vi "Test Initiate.vi"(0 "niDTS BT Rx Test in":refnum<class "niDTS BT Rx Test.lvclass">, 11 "error in (no error)":errorcluster) -> (4 "niDTS BT Rx Test out":refnum<class "niDTS BT Rx Test.lvclass">, 15 "error out":errorcluster)   [LabVIEW 2015, in "niDTS BT.lvlib" / "niDTS BT Rx Test.lvclass"]
uses:
  niDTS BT Rx Test.lvclass
  niDTS BT Rx Test.lvclass/niDTS BT Rx Test.ctl
  Instrument/INSTR RX/niDTS BT INSTR RX.lvclass
  Framework/Dut/Objects/BASE_class/niDTS Dut.lvclass
  Dut/Objects/BASE_class/niDTS BT Dut.lvclass
  niDTS BT.lvlib
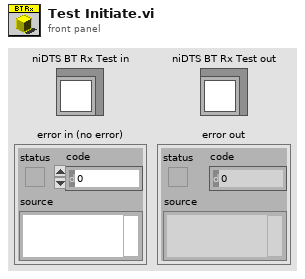
[diagram p1: front panel]
types:
  T1 = typedef "niDTS Framework.lvlib/niDTS Dut INC Handle.ctl" = refnum<data-value>
  T2 = typedef "niDTS BT.lvlib/niDTS BT INC Packet Type.ctl" = enum16{"NULL", "POLL", "FHS", "DM1", "DH1", "HV1", "HV2", "HV3", "EV3", "DV", "AUX1", "DM3", "DH3", "EV4", "EV5", "DM5", "DH5", "LE-TP"}
  T3 = typedef "niDTS BT.lvlib/niDTS BT Dut INC Handle.ctl" = refnum<data-value>
  T4 = typedef "niDTS BT.lvlib/niDTS BT Rx Test INC Results.ctl" = cluster{"Total Packets Received (LE)":i32, "Packets Sent (LE)":dbl, "Good Packets":dbl, "Packet Error Rate (%)":dbl, "Error Bits":u32, "Good Bits":u32, "Total Received Bits":u32, "Bit Error Rate (%)":dbl}
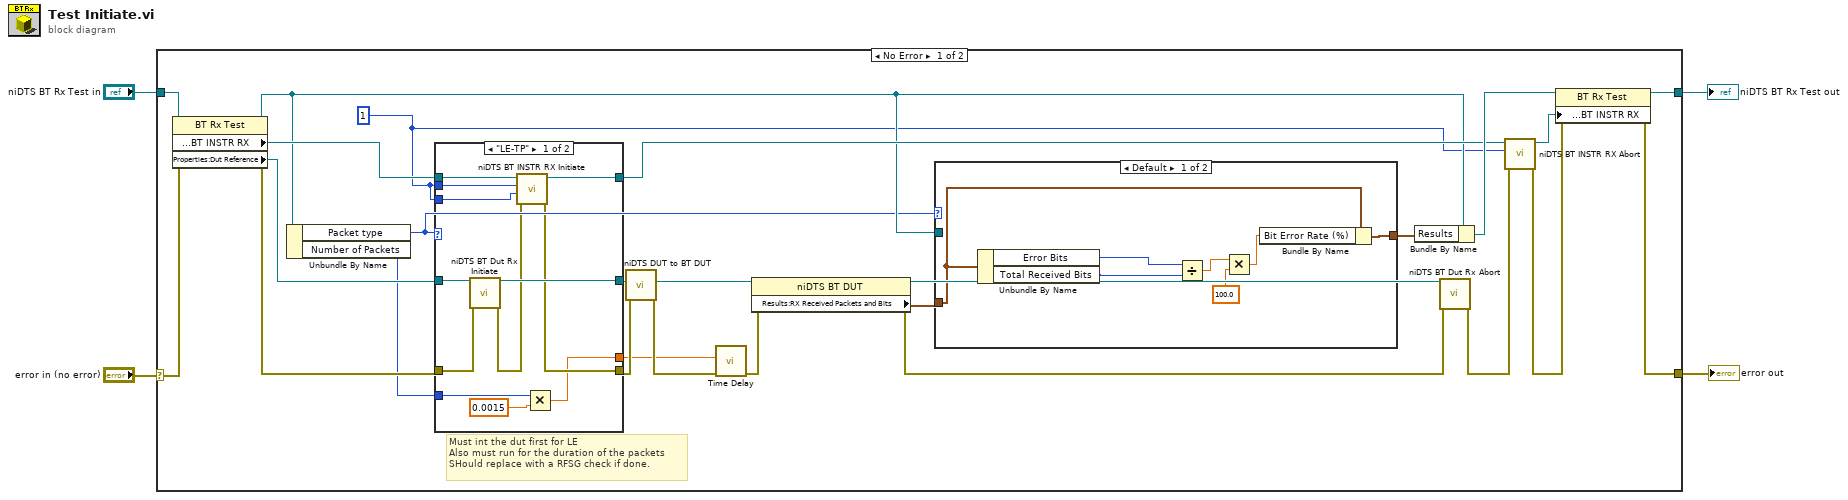
[diagram p0: block diagram]
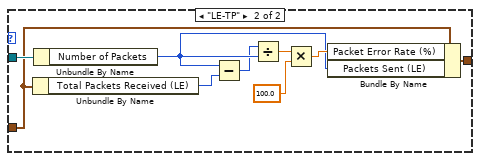
[diagram p2: hidden frame]
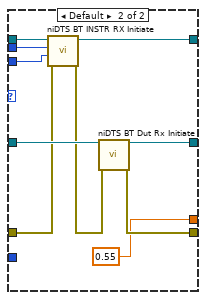
[diagram p3: hidden frame]
diagram:
  n1 = case shown="No Error" "error in (no error)" {
    selector: "error in (no error)" -> [w29 w69]
    tunnel: "niDTS BT Rx Test in" -> [w30 w70]
    tunnel: [w27 w69] -> w3
    tunnel: [w28 w70] -> w2
    frame No Error {
      w5 = 1 ("Driver Instance")
      # "Must int the dut first for LE\nAlso must run for the duration of the packets\nSHould replace with a RFSG check if done."
      n2 = property class="BT Rx Test"(reference=w30, error in=w29) -> (reference out=w12:refnum<class "niDTS BT Rx Test.lvclass">, error out=w21:errorcluster, "Properties:Results:BT INSTR RX"=w14:refnum<class "niDTS BT INSTR RX.lvclass">, "Properties:Dut Reference"=w26:T1)
      n3 = Unbundle By Name(w12) -> ("Packet type"=w9:T2, "Number of Packets"=w6:i32)
      n4 = case shown="\"LE-TP\"" w9 {
        tunnel: w26 -> [w58 w68]
        tunnel: [w57 w67] -> w25
        tunnel: [w51 w66] -> w24
        tunnel: w21 -> [w53 w65]
        tunnel: [w56 w63] -> w13
        tunnel: w5 -> [w55 w62]
        tunnel: w14 -> [w54 w61]
        tunnel: [w47 0.55 ("Delay Time (s)")] -> w7
        tunnel: w6 -> [w50 _]
        tunnel: w5 -> [w48 w59]
        frame "LE-TP" {
          n5 = call "niDTS BT Dut Rx Initiate.vi"("Dut Handle in"=w58, "error in (no error)"=w53) -> ("Dut Handle out"=w57:T1, "error out"=w52:errorcluster)  [unwired: 12 in]
          n6 = call-dynamic "niDTS BT INSTR RX Initiate.vi"("error in (no error)"=w52, "Result Index"=w48, "Driver Instance"=w55, "niDTS BT INSTR RX in"=w54) -> ("error out"=w51:errorcluster, "niDTS BT INSTR RX out"=w56:refnum<class "niDTS BT INSTR RX.lvclass">)  [unwired: 6 in]
          n7 = Multiply(x=w50, y=0.0015 ("Numeric")) -> (x*y=w47:dbl)
        }
        frame Default {
          n8 = call-dynamic "niDTS BT INSTR RX Initiate.vi"("error in (no error)"=w65, "Result Index"=w59, "Driver Instance"=w62, "niDTS BT INSTR RX in"=w61) -> ("error out"=w64:errorcluster, "niDTS BT INSTR RX out"=w63:refnum<class "niDTS BT INSTR RX.lvclass">)  [unwired: 6 in]
          n9 = call "niDTS BT Dut Rx Initiate.vi"("Dut Handle in"=w68, "error in (no error)"=w64) -> ("Dut Handle out"=w67:T1, "error out"=w66:errorcluster)  [unwired: 12 in]
        }
      }
      n10 = call "niDTS DUT to BT DUT.vi"("error in"=w24, "Dut Handle"=w25) -> ("error out"=w20:errorcluster, "BT Dut Handle"=w23:T3)  [unwired: 8 in]
      n11 = call "Time Delay"("error in (no error)"=w20, "Delay Time (s)"=w7) -> ("error out"=w19:errorcluster)  [unwired: 9 in]
      n12 = property class="niDTS BT DUT"(reference=w23, error in=w19) -> (reference out=w8:T3, error out=w18:errorcluster, "Results:RX Received Packets and Bits"=w11:T4)
      n13 = case shown="Default" w9 {
        tunnel: w12 -> [_ w46]
        tunnel: w11 -> [w35 w41]
        tunnel: [w37 w45] -> w10
        frame Default {
          n14 = Unbundle By Name(w35) -> ("Error Bits"=w36:u32, "Total Received Bits"=w34:u32)
          n15 = Divide(x=w36, y=w34) -> (x/y=w33:dbl)
          n16 = Multiply(x=w33, y=100.0) -> (x*y=w32:dbl)
          n17 = Bundle By Name(cluster=w35, "Bit Error Rate (%)"=w32) -> (w37:T4)
        }
        frame "LE-TP" {
          n18 = Unbundle By Name(w41) -> ("Total Packets Received (LE)"=w40:i32)
          n19 = Unbundle By Name(w46) -> ("Number of Packets"=w39:i32)
          n20 = Subtract(x=w39, y=w40) -> (x-y=w38:i32)
          n21 = Divide(x=w38, y=w39) -> (x/y=w44:dbl)
          n22 = Multiply(x=w44, y=100.0) -> (x*y=w43:dbl)
          n23 = Bundle By Name(cluster=w41, "Packet Error Rate (%)"=w43, "Packets Sent (LE)"=w39) -> (w45:T4)
        }
      }
      n24 = Bundle By Name(cluster=w12, "Results"=w10) -> (w22:refnum<class "niDTS BT Rx Test.lvclass">)
      n25 = call "niDTS BT Dut Rx Abort.vi"("BT Dut Handle in"=w8, "error in (no error)"=w18) -> ("error out"=w16:errorcluster)  [unwired: 12 in, 1 out]
      n26 = call-dynamic "niDTS BT INSTR RX Abort.vi"("error in (no error)"=w16, "Driver Instance"=w5, "niDTS BT INSTR RX in"=w13) -> ("error out"=w15:errorcluster, "niDTS BT INSTR RX out"=w17:refnum<class "niDTS BT INSTR RX.lvclass">)  [unwired: 7 in]
      n27 = property class="BT Rx Test"(reference=w22, error in=w15, "Properties:Results:BT INSTR RX"=w17) -> (reference out=w28:refnum<class "niDTS BT Rx Test.lvclass">, error out=w27:errorcluster)
    }
    frame Error {
    }
  }
  "error out" <- w3
  "niDTS BT Rx Test out" <- w2
